vi "Curtin_BuildCursorList.vi"(2 "Allow Drag?":bool, 3 "Fctr":ext[](array[numeric])) -> (0 "Freq Titles":string[](array[string]), 1 "Cursor List":T1(array[cluster]))   [LabVIEW 2022 SP3]
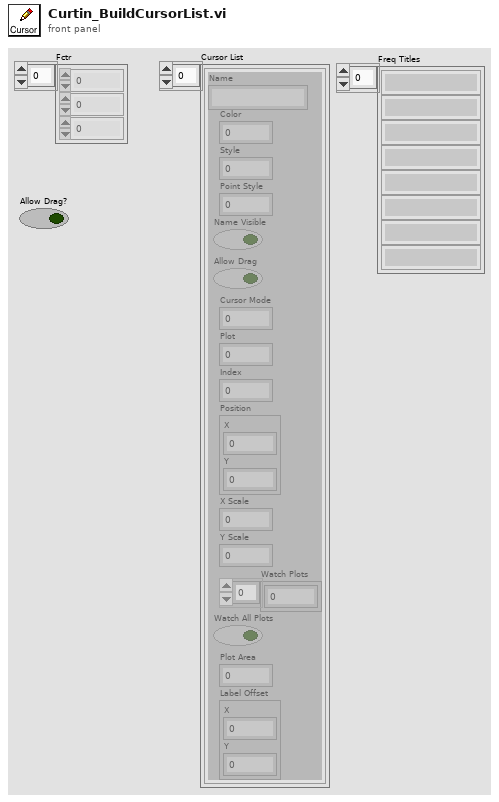
[diagram p1: front panel]
types:
  T1 = cluster{"Name":string, "Color":u32, "Style":u8, "Point Style":u8, "Name Visible":bool, "Allow Drag":bool, "Cursor Mode":u32, "Plot":i32, "Index":i32, "Position":cluster{"X":dbl, "Y":dbl}, "X Scale":u32, "Y Scale":u32, "Watch Plots":i32[], "Watch All Plots":bool, "Plot Area":i32, "Label Offset":cluster{"X":dbl, "Y":dbl}}[]
  T2 = cluster{"Name":string, "Color":u32, "Style":u8, "Point Style":u8, "Name Visible":bool, "Allow Drag":bool, "Cursor Mode":u32, "Plot":i32, "Index":i32, "Position":cluster{"X":dbl, "Y":dbl}, "X Scale":u32, "Y Scale":u32, "Watch Plots":i32[], "Watch All Plots":bool, "Plot Area":i32, "Label Offset":cluster{"X":dbl, "Y":dbl}}
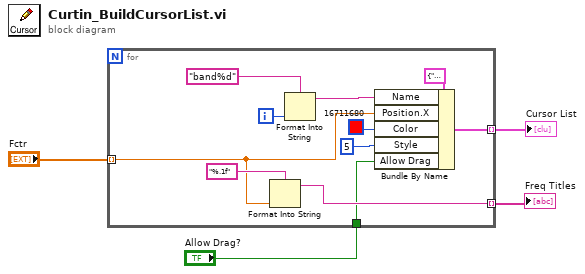
[diagram p0: block diagram]
diagram:
  n1 = for {
    tunnel: "Fctr" -> [w8] mode=indexing
    tunnel: [w14] -> w1 mode=indexing
    tunnel: [w9] -> w2 mode=indexing
    tunnel: "Allow Drag?" -> [w5]
    i -> [w10]
    n2 = Format Into String(format string="%.1f", w8) -> (resulting string=w14:string)  [unwired: 2 in, 1 out]
    n3 = Format Into String(format string="band%d", w10) -> (resulting string=w12:string)  [unwired: 2 in, 1 out]
    n4 = Bundle By Name(cluster=T2 {"Name"="", "Color"=0, "Style"=0, "Point Style"=0, "Name Visible"=FALSE, "Allow Drag"=FALSE, "Cursor Mode"=0, "Plot"=0, "Index"=0, "Position"={"X"=0.0, "Y"=0.0}, "X Scale"=0, "Y Scale"=0, "Watch Plots"=[], "Watch All Plots"=FALSE, "Plot Area"=0, "Label Offset"={"X"=0.0, "Y"=0.0}}, "Name"=w12, "Position.X"=w8, "Color"=u32 16711680, "Style"=u8 5 ("Cursor.Cursor Style"), "Allow Drag"=w5) -> (w9:T2)
  }
  "Cursor List" <- w2
  "Freq Titles" <- w1
